vi "can fd bitrate constant (sae j2284-4).vi"() -> (0 "bitrate":T1={"clock frequency"=enum."CLOCK_24MHz", "nominal bitrate"={"bitrate prescaler"=0, "time segment 1"=0, "time segment 2"=0, "sync jump width"=0}, "data bitrate"={"bitrate prescaler"=0, "time segment 1"=0, "time segment 2"=0, "sync jump width"=0}})   [LabVIEW 2024, in "atsj peakcan basic.lvlib"]
doc: "SAE J2284-4: High-Speed CAN (HSC) for Vehicle Applications at 500 kbps with CAN FD Data at 2 Mbps.\n\nCopyright (c) 2025 ATSJ (www.atsj.eu)"
uses:
  atsj peakcan basic.lvlib
  fd bitrate.ctl
  clock frequency.ctl
  fd bitrate parameters.ctl
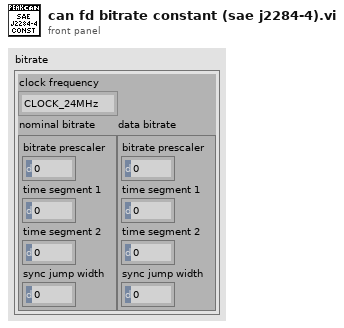
[diagram p1: front panel]
types:
  T1 = typedef "atsj peakcan basic.lvlib/fd bitrate.ctl" = cluster{"clock frequency":T2, "nominal bitrate":T3, "data bitrate":T3}
  T2 = typedef "atsj peakcan basic.lvlib/clock frequency.ctl" = enum16{"CLOCK_80MHz", "CLOCK_60MHz", "CLOCK_40MHz", "CLOCK_30MHz", "CLOCK_24MHz", "CLOCK_20MHz"}
  T3 = typedef "atsj peakcan basic.lvlib/fd bitrate parameters.ctl" = cluster{"bitrate prescaler":u16, "time segment 1":u16, "time segment 2":u16, "sync jump width":u16}
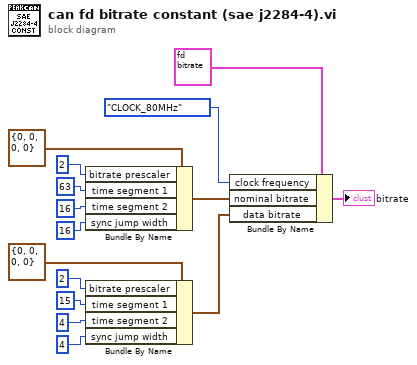
[diagram p0: block diagram]
diagram:
  n1 = Bundle By Name(cluster=T3 {"bitrate prescaler"=0, "time segment 1"=0, "time segment 2"=0, "sync jump width"=0}, "bitrate prescaler"=u16 2, "time segment 1"=u16 63, "time segment 2"=u16 16, "sync jump width"=u16 16) -> (w12:T3)
  n2 = Bundle By Name(cluster=T3 {"bitrate prescaler"=0, "time segment 1"=0, "time segment 2"=0, "sync jump width"=0}, "bitrate prescaler"=u16 2, "time segment 1"=u16 15, "time segment 2"=u16 4, "sync jump width"=u16 4) -> (w11:T3)
  n3 = Bundle By Name(cluster=T1 {"clock frequency"=enum."CLOCK_24MHz", "nominal bitrate"={"bitrate prescaler"=0, "time segment 1"=0, "time segment 2"=0, "sync jump width"=0}, "data bitrate"={"bitrate prescaler"=0, "time segment 1"=0, "time segment 2"=0, "sync jump width"=0}}, "clock frequency"=clock_frequency."CLOCK_80MHz", "nominal bitrate"=w12, "data bitrate"=w11) -> (→"bitrate":T1)
